vi "MGCC_FntStaMach_threephase_figureplot.vi"() -> (0 "appended array":cluster{dbl[], dbl[]}[](array[cluster]))   [LabVIEW 2016]
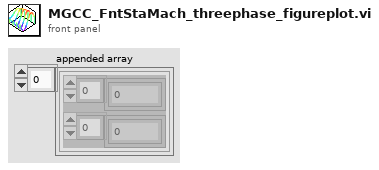
[diagram p1: front panel]
types:
  T1 = cluster{"V_node":cdb[][], "P_node":cdb[][], "I_node":cdb[][], "NumN":dbl, "NumL":dbl, "Ybus":cdb[][], "sspn":dbl[][], "ssqn":dbl[][], "ssvn":dbl[][], "SlackBus":dbl, "Topology":dbl[][]}
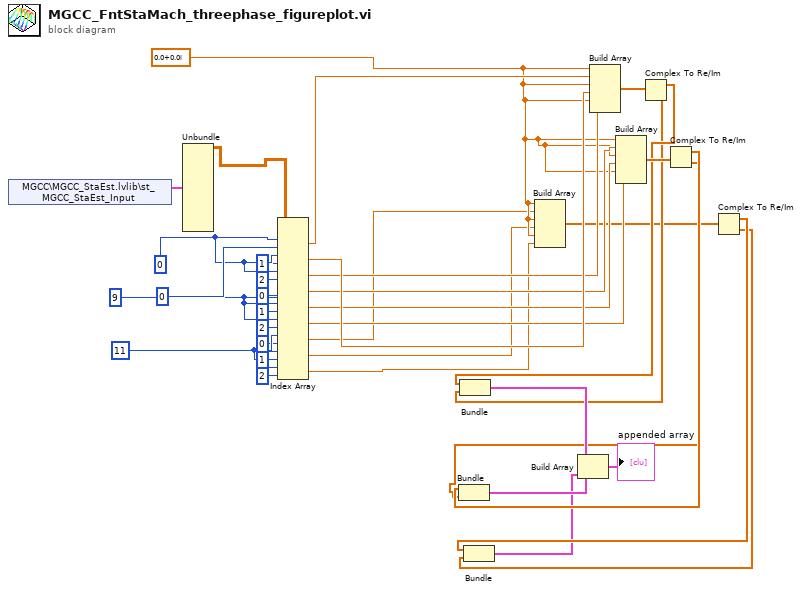
[diagram p0: block diagram]
diagram:
  w12 = 11 ("index (row)")
  w29 = 9 ("index (row)")
  w35 = 0 ("disabled index (row)")
  w8 = csg 0.0+0.0i ("element")
  n1 = shared-variable "MGCC\\MGCC_StaEst.lvlib\\st_MGCC_StaEst_Input"() -> (w37:T1)  [unwired: 1 in, 1 out]
  n2 = Unbundle(w37) -> ("V_node"=w20:cdb[][])  [unwired: 10 out]
  n3 = Index Array(array=w20, index (row) #1=w35, index (col) #1=0 ("disabled index (col)"), index (row) #2=w35, index (col) #2=1 ("disabled index (col)"), index (row) #3=w35, index (col) #3=2 ("disabled index (col)"), index (row) #4=w29, index (col) #4=0 ("disabled index (col)"), index (row) #5=w29, index (col) #5=1 ("disabled index (col)"), index (row) #6=w29, index (col) #6=2 ("disabled index (col)"), index (row) #7=w12, index (col) #7=0 ("disabled index (col)"), index (row) #8=w12, index (col) #8=1 ("disabled index (col)"), index (row) #9=w12, index (col) #9=2 ("disabled index (col)")) -> (element #1=w31:cdb, element #2=w32:cdb, element #3=w30:cdb, element #4=w25:cdb, element #5=w24:cdb, element #6=w23:cdb, element #7=w7:cdb, element #8=w6:cdb, element #9=w5:cdb)
  n4 = Build Array(w8, w7, w8, w6, w8, w5) -> (w4:cdb[])
  n5 = Build Array(w8, w31, w8, w32, w8, w30) -> (w19:cdb[])
  n6 = Build Array(w8, w25, w8, w24, w8, w23) -> (w18:cdb[])
  n7 = Complex To Re/Im(x + iy=w19) -> (x=w17:dbl[], y=w16:dbl[])
  n8 = Bundle(w17, w16) -> (w22:cluster{dbl[], dbl[]})  [unwired: 1 in]
  n9 = Complex To Re/Im(x + iy=w18) -> (x=w15:dbl[], y=w14:dbl[])
  n10 = Bundle(w15, w14) -> (w21:cluster{dbl[], dbl[]})  [unwired: 1 in]
  n11 = Complex To Re/Im(x + iy=w4) -> (x=w3:dbl[], y=w2:dbl[])
  n12 = Bundle(w3, w2) -> (w1:cluster{dbl[], dbl[]})  [unwired: 1 in]
  n13 = Build Array(w22, w21, w1) -> (→"appended array":cluster{dbl[], dbl[]}[])
